vi "LIN_Message analysis.vi"(10 "Frame":T6, 11 "Value in":string[][](array[string])) -> (3 "Value out":string[][](array[string]))   [LabVIEW 2014]
uses:
  Typedef/TDBFrameProperties.ctl
  Typedef/CAN/TCANSignal.ctl
  Typedef/LIN/TLINSignal.ctl
  Typedef/FlexRay/TFlexRaySignal.ctl
  Typedef/TDBSignalProperties.ctl
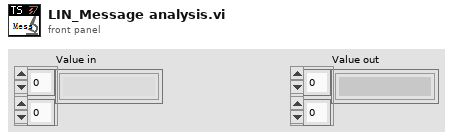
[diagram p1: front panel]
types:
  T1 = typedef "TDBFrameProperties.ctl" = cluster{"FDBIndex":i32, "FECUIndex":i32, "FFrameIndex":i32, "FIsTx":u8, "FReserved1":u8, "FCycleTimeMs":u16, "TSignalType":i32, "FCANIsDataFrame":u8, "FCANIsStdFrame":u8, "FCANIsEdl":u8, "FCANIsBrs":u8, "FCANIdentifier":i32, "FCANDLC":i32, "FCANDataBytes":i32, "FLINIdentifier":i32, "FLINDLC":i32, "FFRChannelMask":u8, "FFRBaseCycle":u8, "FFRCycleRepetition":u8, "FFRIsStartupFrame":u8, "FFRSlotId":u16, "FFRDLC":u16, "FFRCycleMask":u64, "FSignalCount":i32, "FName":cluster{"数值":u64, "数值 2":u64, "数值 3":u64, "数值 4":u64, "数值 5":u64, "数值 6":u64, "数值 7":u64, "数值 8":u64, "数值 9":u64, "数值 10":u64, "数值 11":u64, "数值 12":u64, "数值 13":u64, "数值 14":u64, "数值 15":u64, "数值 16":u64, "数值 17":u64, "数值 18":u64, "数值 19":u64, "数值 20":u64, "数值 21":u64, "数值 22":u64, "数值 23":u64, "数值 24":u64, "数值 25":u64, "数值 26":u64, "数值 27":u64, "数值 28":u64, "数值 29":u64, "数值 30":u64, "数值 31":u64, "数值 32":u64, "数值 33":u64, "数值 34":u64, "数值 35":u64, "数值 36":u64, "数值 37":u64, "数值 38":u64, "数值 39":u64, "数值 40":u64, "数值 41":u64, "数值 42":u64, "数值 43":u64, "数值 44":u64, "数值 45":u64, "数值 46":u64, "数值 47":u64, "数值 48":u64, "数值 49":u64, "数值 50":u64, "数值 51":u64, "数值 52":u64, "数值 53":u64, "数值 54":u64, "数值 55":u64, "数值 56":u64, "数值 57":u64, "数值 58":u64, "数值 59":u64, "数值 60":u64, "数值 61":u64, "数值 62":u64, "数值 63":u64, "数值 64":u64}, "FComment":cluster{"数值":u64, "数值 2":u64, "数值 3":u64, "数值 4":u64, "数值 5":u64, "数值 6":u64, "数值 7":u64, "数值 8":u64, "数值 9":u64, "数值 10":u64, "数值 11":u64, "数值 12":u64, "数值 13":u64, "数值 14":u64, "数值 15":u64, "数值 16":u64, "数值 17":u64, "数值 18":u64, "数值 19":u64, "数值 20":u64, "数值 21":u64, "数值 22":u64, "数值 23":u64, "数值 24":u64, "数值 25":u64, "数值 26":u64, "数值 27":u64, "数值 28":u64, "数值 29":u64, "数值 30":u64, "数值 31":u64, "数值 32":u64, "数值 33":u64, "数值 34":u64, "数值 35":u64, "数值 36":u64, "数值 37":u64, "数值 38":u64, "数值 39":u64, "数值 40":u64, "数值 41":u64, "数值 42":u64, "数值 43":u64, "数值 44":u64, "数值 45":u64, "数值 46":u64, "数值 47":u64, "数值 48":u64, "数值 49":u64, "数值 50":u64, "数值 51":u64, "数值 52":u64, "数值 53":u64, "数值 54":u64, "数值 55":u64, "数值 56":u64, "数值 57":u64, "数值 58":u64, "数值 59":u64, "数值 60":u64, "数值 61":u64, "数值 62":u64, "数值 63":u64, "数值 64":u64}}
  T2 = typedef "TDBSignalProperties.ctl" = cluster{"FDBIndex":i32, "FECUIndex":i32, "FFrameIndex":i32, "FSignalIndex":i32, "FIsTx":u8, "FReserved1":u8, "FReserved2":u8, "FReserved3":u8, "TSignalType":i32, "TCANSignal":T3, "TLINSignal":T4, "TFlexRaySignal":T5, "FParentFrameId":i32, "FInitValue":dbl, "FName":cluster{"数值":u64, "数值 2":u64, "数值 3":u64, "数值 4":u64, "数值 5":u64, "数值 6":u64, "数值 7":u64, "数值 8":u64, "数值 9":u64, "数值 10":u64, "数值 11":u64, "数值 12":u64, "数值 13":u64, "数值 14":u64, "数值 15":u64, "数值 16":u64, "数值 17":u64, "数值 18":u64, "数值 19":u64, "数值 20":u64, "数值 21":u64, "数值 22":u64, "数值 23":u64, "数值 24":u64, "数值 25":u64, "数值 26":u64, "数值 27":u64, "数值 28":u64, "数值 29":u64, "数值 30":u64, "数值 31":u64, "数值 32":u64, "数值 33":u64, "数值 34":u64, "数值 35":u64, "数值 36":u64, "数值 37":u64, "数值 38":u64, "数值 39":u64, "数值 40":u64, "数值 41":u64, "数值 42":u64, "数值 43":u64, "数值 44":u64, "数值 45":u64, "数值 46":u64, "数值 47":u64, "数值 48":u64, "数值 49":u64, "数值 50":u64, "数值 51":u64, "数值 52":u64, "数值 53":u64, "数值 54":u64, "数值 55":u64, "数值 56":u64, "数值 57":u64, "数值 58":u64, "数值 59":u64, "数值 60":u64, "数值 61":u64, "数值 62":u64, "数值 63":u64, "数值 64":u64}, "FComment":cluster{"数值":u64, "数值 2":u64, "数值 3":u64, "数值 4":u64, "数值 5":u64, "数值 6":u64, "数值 7":u64, "数值 8":u64, "数值 9":u64, "数值 10":u64, "数值 11":u64, "数值 12":u64, "数值 13":u64, "数值 14":u64, "数值 15":u64, "数值 16":u64, "数值 17":u64, "数值 18":u64, "数值 19":u64, "数值 20":u64, "数值 21":u64, "数值 22":u64, "数值 23":u64, "数值 24":u64, "数值 25":u64, "数值 26":u64, "数值 27":u64, "数值 28":u64, "数值 29":u64, "数值 30":u64, "数值 31":u64, "数值 32":u64, "数值 33":u64, "数值 34":u64, "数值 35":u64, "数值 36":u64, "数值 37":u64, "数值 38":u64, "数值 39":u64, "数值 40":u64, "数值 41":u64, "数值 42":u64, "数值 43":u64, "数值 44":u64, "数值 45":u64, "数值 46":u64, "数值 47":u64, "数值 48":u64, "数值 49":u64, "数值 50":u64, "数值 51":u64, "数值 52":u64, "数值 53":u64, "数值 54":u64, "数值 55":u64, "数值 56":u64, "数值 57":u64, "数值 58":u64, "数值 59":u64, "数值 60":u64, "数值 61":u64, "数值 62":u64, "数值 63":u64, "数值 64":u64}}
  T3 = typedef "TCANSignal.ctl" = cluster{"FCANSgnType":u8, "FIsIntel":u8, "FStartBit":i32, "FLength":i32, "FFactor":dbl, "FOffset":dbl}
  T4 = typedef "TLINSignal.ctl" = cluster{"FLINSgnType":u8, "FIsIntel":u8, "FStartBit":i32, "FLength":i32, "FFactor":dbl, "FOffset":dbl}
  T5 = typedef "TFlexRaySignal.ctl" = cluster{"FFRSgnType":u8, "FCompuMethod":u8, "FReserved":u8, "FIsIntel":u8, "FStartBit":i32, "FUpdateBit":i32, "FLength":i32, "FFactor":dbl, "FOffset":dbl, "FActualStartBit":i32, "FActualUpdateBit":i32}
  T6 = cluster{"Frame_Properties":T1, "signal_array":T2[]}
  T7 = cluster{"数值":u64, "数值 2":u64, "数值 3":u64, "数值 4":u64, "数值 5":u64, "数值 6":u64, "数值 7":u64, "数值 8":u64, "数值 9":u64, "数值 10":u64, "数值 11":u64, "数值 12":u64, "数值 13":u64, "数值 14":u64, "数值 15":u64, "数值 16":u64, "数值 17":u64, "数值 18":u64, "数值 19":u64, "数值 20":u64, "数值 21":u64, "数值 22":u64, "数值 23":u64, "数值 24":u64, "数值 25":u64, "数值 26":u64, "数值 27":u64, "数值 28":u64, "数值 29":u64, "数值 30":u64, "数值 31":u64, "数值 32":u64, "数值 33":u64, "数值 34":u64, "数值 35":u64, "数值 36":u64, "数值 37":u64, "数值 38":u64, "数值 39":u64, "数值 40":u64, "数值 41":u64, "数值 42":u64, "数值 43":u64, "数值 44":u64, "数值 45":u64, "数值 46":u64, "数值 47":u64, "数值 48":u64, "数值 49":u64, "数值 50":u64, "数值 51":u64, "数值 52":u64, "数值 53":u64, "数值 54":u64, "数值 55":u64, "数值 56":u64, "数值 57":u64, "数值 58":u64, "数值 59":u64, "数值 60":u64, "数值 61":u64, "数值 62":u64, "数值 63":u64, "数值 64":u64}
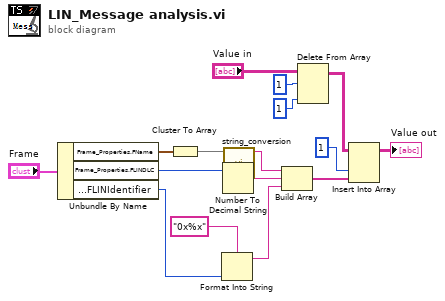
[diagram p0: block diagram]
diagram:
  n1 = Unbundle By Name("Frame") -> ("Frame_Properties.FName"=w6:T7, "Frame_Properties.FLINDLC"=w5:i32, "Frame_Properties.FLINIdentifier"=w4:i32)
  n2 = Cluster To Array(cluster=w6) -> (array=w2:u64[])
  n3 = Format Into String(format string="0x%x", w4) -> (resulting string=w9:string)  [unwired: 2 in, 1 out]
  n4 = Number To Decimal String(number=w5) -> (decimal integer string=w8:string)  [unwired: 1 in]
  n5 = call "string_conversion.vi"("FName"=w2) -> ("string"=w1:string)  [unwired: 10 in]
  n6 = Build Array(w1, w8, w9) -> (w15:string[])
  n7 = Delete From Array(array="Value in", length=1 ("disabled index (col)"), index (col)=1 ("disabled index (col)")) -> (array with subset deleted=w13:string[][])  [unwired: 1 in, 1 out]
  n8 = Insert Into Array(array=w13, index (col)=1 ("disabled index (col)"), new element=w15) -> (→"Value out":string[][])  [unwired: 1 in]
